vi "BLM control.vi"(2 "Point #":i32, 4 "Parameters":dbl[](array[numeric]) format="%.3e", 5 "Instrument Address":refnum<visa-resource-name>) -> (0 "Stop":bool, 1 "Data Out":dbl[](array[numeric]) format="%.2f")   [LabVIEW 2019]
doc: "Moves the stepper moter an appropriate amount based on the point number, step size and final position.\nScott Hannahs, NHMFL, March 1999"
uses:
  Serial Instruments/Serial Support VISA.llb/Serial Actions.ctl
panel:
  in  "Motor Address":string="0"
  in  "error in (no error)":errorcluster
  out "Starting Position":dbl format="%.2f"
  # "Motor Number"
  # "Step Size"
  # "Final Position"
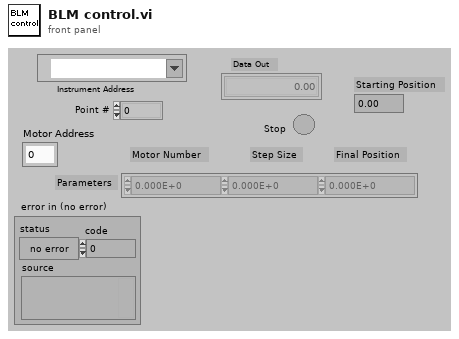
[diagram p1: front panel]
types:
  T1 = cluster{"Parameters[0]":dbl, "Parameters[1]":dbl, "Parameters[2]":dbl}
  T2 = typedef "Serial Actions.ctl" = enum16{"Init", "Break", "Clear Buffer", "Write", "Read", "N Bytes", "Lock", "Unlock", "Close"}
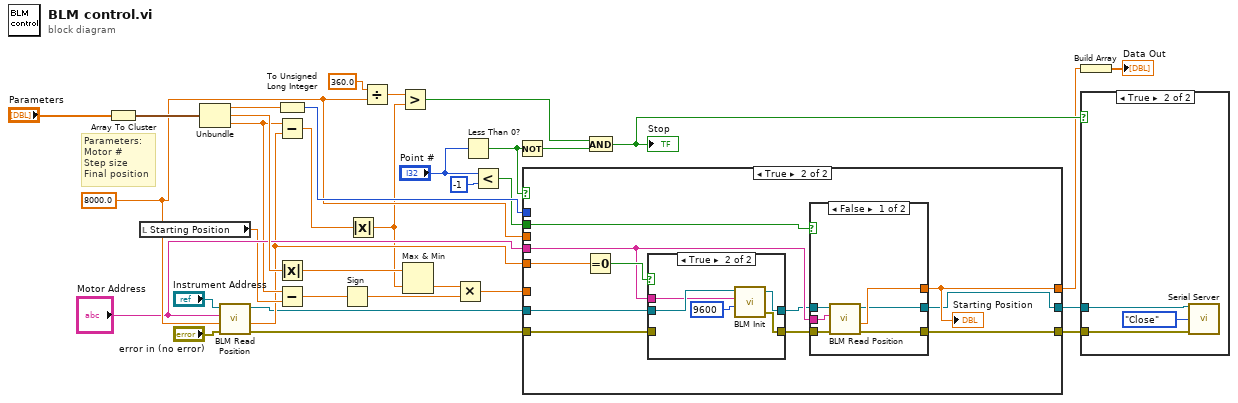
[diagram p0: block diagram]
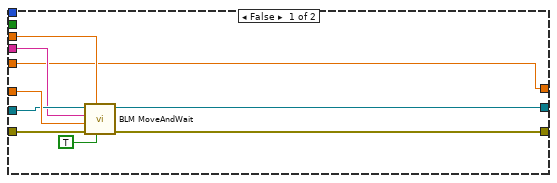
[diagram p3: hidden frame]
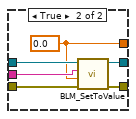
[diagram p5: hidden frame]
diagram:
  w15 = 8000.0 ("Steps/rot")
  # "Parameters:\nMotor #\nStep size\nFinal position"
  n1 = Array To Cluster(array="Parameters") -> (cluster=w33:T1)
  n2 = local read "Starting Position"() -> (w11:dbl)
  n3 = Unbundle(w33) -> ("Parameters[0]"=w32:dbl, "Parameters[1]"=w25:dbl, "Parameters[2]"=w8:dbl)
  n4 = call "BLM Read Position.vi"("error in (no error)"="error in (no error)", "Steps/rot"=w15, "Motor Address"="Motor Address", "Port Address"="Instrument Address") -> ("error out"=w13:errorcluster, "Response"=w7:dbl, "Port Address Out"=w1:refnum<visa-resource-name>)  [unwired: 1 out]
  n5 = To Unsigned Long Integer(number=w32) -> (unsigned 32bit integer=w29:u32)
  n6 = Subtract(x=w8, y=w7) -> (x-y=w6:dbl)
  n7 = Absolute Value(x=w25) -> (abs(x)=w5:dbl)
  n8 = Subtract(x=w8, y=w11) -> (x-y=w10:dbl)
  n9 = Sign(1:w10) -> (0:w24:dbl)
  n10 = Absolute Value(x=w6) -> (abs(x)=w4:dbl)
  n11 = Divide(x=360.0, y=w15) -> (x/y=w3:dbl)
  n12 = Greater?(x=w3, y=w4) -> (0:w22:bool)
  n13 = Max & Min(x=w5, y=w4) -> (min(x,y)=w9:dbl)  [unwired: 1 out]
  n14 = Multiply(x=w9, y=w24) -> (x*y=w19:dbl)
  n15 = Less Than 0?(x="Point #") -> (x < 0?=w21:bool)
  n16 = Less?(x="Point #", y=-1) -> (x < y?=w26:bool)
  n17 = Not(x=w21) -> (.not. x?=w20:bool)
  n18 = case shown="True" w21 {
    tunnel: w1 -> [w40 w50]
    tunnel: [w35 w44] -> w30
    tunnel: w29 -> [_ _]
    tunnel: [w43 w54] -> w17
    tunnel: w26 -> [_ w53]
    tunnel: w19 -> [w42 _]
    tunnel: w15 -> [w38 _]
    tunnel: "Motor Address" -> [w39 w49]
    tunnel: [w37 w48] -> w18
    tunnel: w7 -> [w37 w47]
    tunnel: w13 -> [w36 w46]
    frame False {
      n19 = call "BLM MoveAndWait.vi"("Mode IS:"=TRUE ("Mode"), "Steps/rot"=w38, "error in (no error)"=w36, "Position / Distance"=w42, "Motor Address"=w39, "Instrument Address"=w40) -> ("error out"=w43:errorcluster, "PORT Address 2"=w35:refnum<visa-resource-name>)  [unwired: 2 in]
    }
    frame True {
      n20 = Equal To 0?(x=w47) -> (x = 0?=w51:bool)
      n21 = case shown="True" w51 {
        tunnel: w50 -> [w55 w60]
        tunnel: [w56 w59] -> w52
        tunnel: w49 -> [_ w58]
        tunnel: w46 -> [w56 _]
        tunnel: [w55 w57] -> w45
        frame False {
        }
        frame True {
          n22 = call "BLM Init.vi"("Baud Rate"=u32 9600, "Motor Address"=w58, "Port Address"=w60) -> ("error out"=w59:errorcluster, "Port Address Out"=w57:refnum<visa-resource-name>)  [unwired: 1 in, 1 out]
        }
      }
      n23 = case shown="False" w53 {
        tunnel: w45 -> [w67 w73]
        tunnel: [w66 w72] -> w54
        tunnel: [w65 w69] -> w48
        tunnel: w52 -> [w64 w71]
        tunnel: w49 -> [w63 w70]
        tunnel: [w62 w68] -> w44
        frame False {
          n24 = call "BLM Read Position.vi"("error in (no error)"=w64, "Motor Address"=w63, "Port Address"=w67) -> ("error out"=w66:errorcluster, "Response"=w65:dbl, "Port Address Out"=w62:refnum<visa-resource-name>)  [unwired: 1 in, 1 out]
        }
        frame True {
          w69 = 0.0
          n25 = call "BLM_SetToValue.vi"("error in (no error)"=w71, "Position"=w69, "Motor Address"=w70, "Port Address"=w73) -> ("error out"=w72:errorcluster, "Port Address Out"=w68:refnum<visa-resource-name>)  [unwired: 2 in]
        }
      }
      "Starting Position" <- w48
    }
  }
  n26 = And(x=w22, y=w20) -> (x .and. y?=w23:bool)
  "Stop" <- w23
  n27 = Build Array(w18) -> (→"Data Out":dbl[])
  n28 = case shown="True" w23 {
    tunnel: w30 -> [_ w75]
    tunnel: w17 -> [_ w74]
    frame False {
    }
    frame True {
      n29 = call "Serial Server.vi"("VISA Resource Name"=w75, "Action"=Serial_Actions."Close", "error in (no error)"=w74) -> ()  [unwired: 8 in, 5 out]
    }
  }
